vi "GV_YscaleDeletePoint.vi"(7 "Move?":bool, 8 "error in (no error)":errorcluster, 9 "Pos":cluster{"x":i16, "y":i16}, 10 "Plot in":picture, 11 "Gviewer in":refnum<class "Gviewer.lvclass">) -> (0 "error out":errorcluster, 2 "Plot out":picture, 3 "Gviewer out":refnum<class "Gviewer.lvclass">)   [LabVIEW 2020, in "Sgraph_lib_V1.lvlib" / "Gviewer.lvclass"]
doc: "Andre Koelewijn,11 aug 2021\n\nFocus Y-scale if selected"
uses:
  Gviewer.lvclass
  <vilib>/Utility/miscctls.llb/LVPoint32TypeDef.ctl
  Gviewer.lvclass/Gviewer.ctl
panel:
  in  "Coords":T1
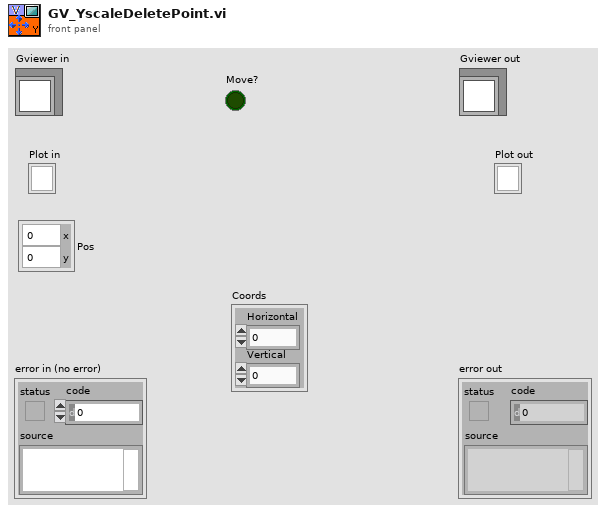
[diagram p1: front panel]
types:
  T1 = typedef "LVPoint32TypeDef.ctl" = cluster{"Horizontal":i32, "Vertical":i32}
  T2 = cluster{"left":i16, "top":i16, "right":i16, "bottom":i16}
  T3 = cluster{"Width":i16, "Style":enum32{"Solid", "Dash", "Dot", "DashDot", "DashDotDot"}}
  T4 = typedef "Sgraph_lib_V1.lvlib/Gviewer.lvclass/YgraphDef.ctl" = cluster{"Plot":i32, "X(%)":dbl}
  T5 = typedef "LVRectTypeDef.ctl" = cluster{"Left":i16, "Top":i16, "Right":i16, "Bottom":i16}
  T6 = cluster{"data":dbl[], "max":dbl[], "min":dbl[], "Status":u32[]}[]
  T7 = typedef "Sgraph_lib_V1.lvlib/Gviewer.lvclass/Typedef_SelProperties.ctl" = cluster{"Color":u32, "LineType":T8, "max":dbl, "min":dbl}
  T8 = typedef "Sgraph_lib_V1.lvlib/Gviewer.lvclass/Typedef_LineType.ctl" = enum16{"num_bare", "num_MinMax_Area", "num_MinMax_Lines", "num_MinMax_Forfor", "num_Max_Area", "num_Max_Line", "num_Max_Forfor", "num_Min_Area", "num_Min_Line", "num_Min_Fosfor", "Boolean_Line_01", "Boolean_Area_01", "Boolean_Fosfor_01", "Boolean_Line_TF", "Boolean_Area_TF", "Boolean_Fosfor_TF", "Boolean_OnOff_Line", "Boolean_OnOff_Area", "Boolean_OnOff_Fosfor", "Boolean_spare", "StringEvent_Line", "StringEvent_TimeLine"}
  T9 = cluster{"data":dbl[], "max":dbl[], "min":dbl[], "Status":u32[]}
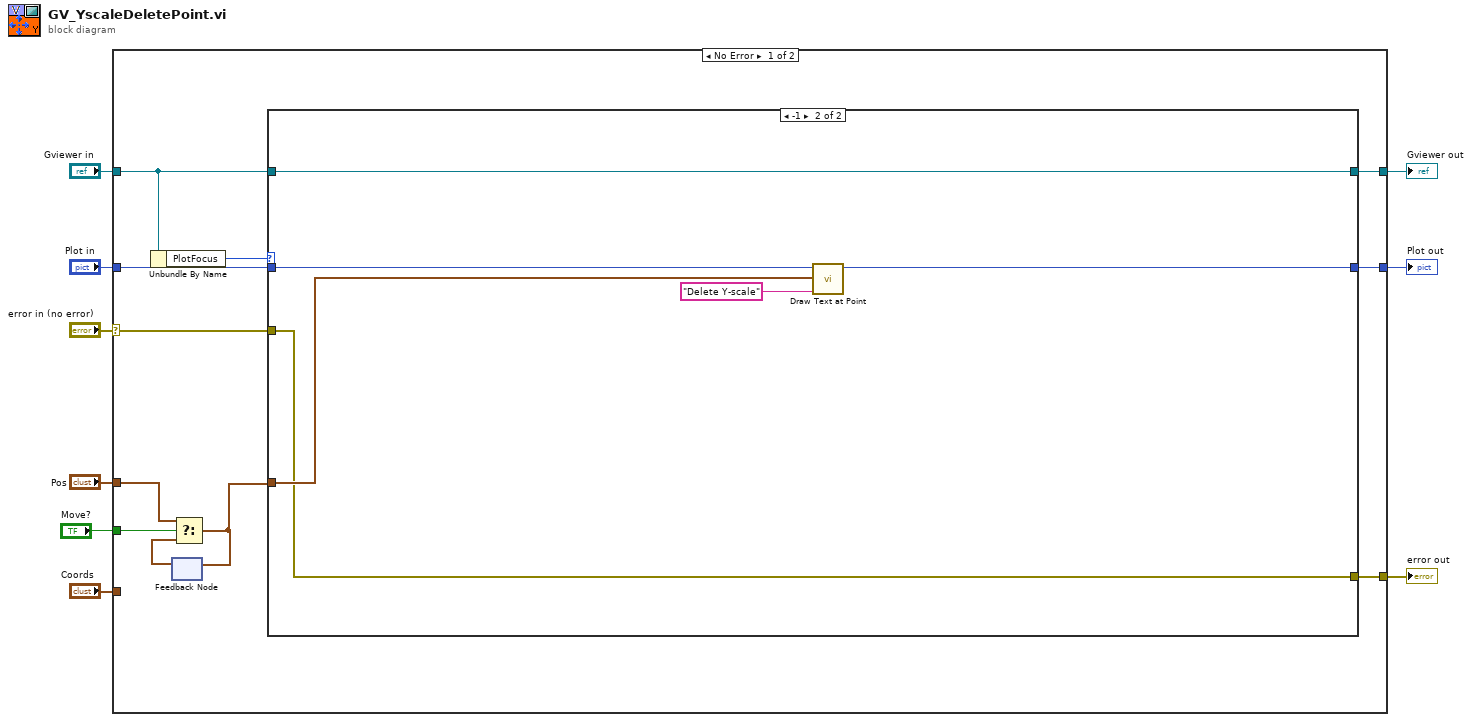
[diagram p0: block diagram]
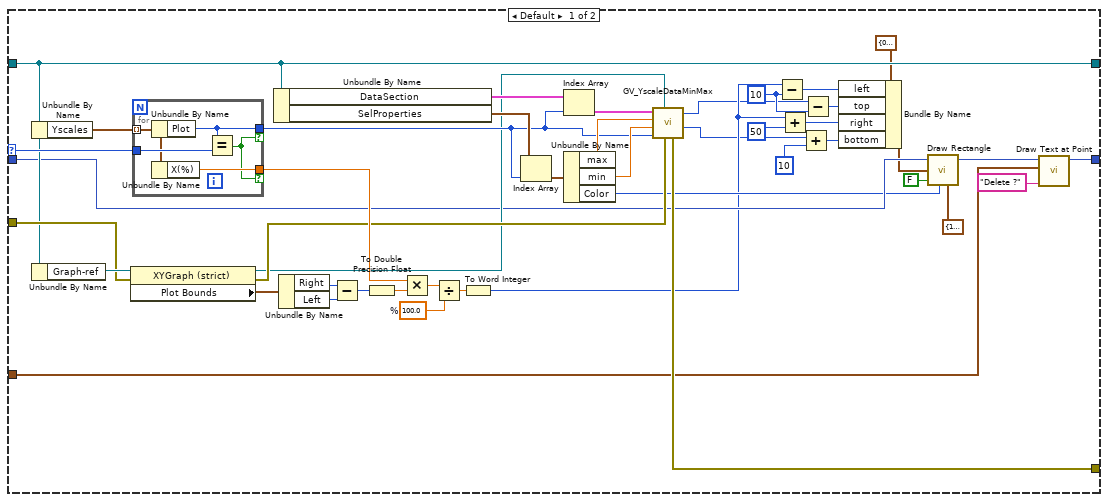
[diagram p2: hidden frame]
diagram:
  n1 = case shown="No Error" "error in (no error)" {
    selector: "error in (no error)" -> [w18 w77]
    tunnel: [w15 w77] -> w8
    tunnel: [w17 w76] -> w6
    tunnel: "Gviewer in" -> [w19 w76]
    tunnel: "Coords" -> [_ _]
    tunnel: [w16 _] -> w4
    tunnel: "Pos" -> [w10 _]
    tunnel: "Plot in" -> [w14 _]
    tunnel: "Move?" -> [w13 _]
    frame No Error {
      n2 = Unbundle By Name(w19) -> ("PlotFocus"=w20:i32)
      n3 = feedback #1() -> (w12:cluster{"x":i16, "y":i16})  [unwired: 1 in]
      n4 = Select(t=w10, s=w13, f=w12) -> (s? t:f=w11:cluster{"x":i16, "y":i16})
      n5 = feedback-in #1(w11) -> ()
      n6 = case shown="-1" w20 {
        selector: w20 -> [w63 _]
        tunnel: [w37 w75] -> w16
        tunnel: w11 -> [w36 w73]
        tunnel: [w43 w72] -> w15
        tunnel: w18 -> [w53 w72]
        tunnel: w19 -> [w50 w71]
        tunnel: [w50 w71] -> w17
        tunnel: w14 -> [w40 w70]
        frame Default {
          w27 = i16 10 ("y")
          w59 = 100.0  # %
          n7 = Unbundle By Name(w50) -> ("Yscales"=w64:T4[])
          n8 = Unbundle By Name(w50) -> ("Graph-ref"=w54:refnum<vi>)
          n9 = property class="XYGraph (strict)"(reference=w54, error in=w53) -> (reference out=w41:refnum<vi>, error out=w44:errorcluster, "Plot Bounds"=w52:T5)
          n10 = for {
            tunnel: w64 -> [w67] mode=indexing
            tunnel: [w68] -> w42 if=w65
            tunnel: w63 -> [w69]
            tunnel: [w66] -> w56 if=w65
            n11 = Unbundle By Name(w67) -> ("Plot"=w68:i32)
            n12 = Unbundle By Name(w67) -> ("X(%)"=w66:dbl)
            n13 = Equal?(x=w68, y=w69) -> (x = y?=w65:bool)
          }
          n14 = Unbundle By Name(w50) -> ("DataSection"=w48:T6, "SelProperties"=w49:T7[])
          n15 = Unbundle By Name(w52) -> ("Right"=w62:i16, "Left"=w61:i16)
          n16 = Subtract(x=w62, y=w61) -> (x-y=w55:i16)
          n17 = To Double Precision Float(number=w55) -> (double precision float=w57:dbl)
          n18 = Multiply(x=w56, y=w57) -> (x*y=w60:dbl)
          n19 = Divide(x=w60, y=w59) -> (x/y=w58:dbl)
          n20 = To Word Integer(number=w58) -> (16bit integer=w29:i16)
          n21 = Index Array(array=w49, index=w42) -> (element=w51:T7)
          n22 = Index Array(array=w48, index=w42) -> (element=w47:T9)
          n23 = Unbundle By Name(w51) -> ("max"=w46:dbl, "min"=w45:dbl, "Color"=w35:u32)
          n24 = call "GV_YscaleDataMinMax.vi"("error in (no error)"=w44, "Graph-ref"=w41, "Plot"=w42, "Scale-min"=w45, "Scale-max"=w46, "PAQ-data"=w47) -> ("Coord-min"=w21:i32, "Coord-max"=w22:i32, "error out"=w43:errorcluster)  [unwired: 1 in, 2 out]
          n25 = Subtract(x=w29, y=w27) -> (x-y=w30:i16)
          n26 = Add(x=w29, y=i16 50) -> (x+y=w25:i16)
          n27 = Add(x=w21, y=i16 10) -> (x+y=w23:i32)
          n28 = Subtract(x=w22, y=w27) -> (x-y=w26:i32)
          n29 = Bundle By Name(cluster=T2 {"left"=0, "top"=0, "right"=0, "bottom"=0} ("rect"), "left"=w30, "top"=w26, "right"=w25, "bottom"=w23) -> (w32:T2)
          n30 = call <vilib>:"Draw Rectangle.vi"("picture"=w40, "rect"=w32, "fill?(F)"=FALSE, "color(black)"=w35, "pen"=T3 {"Width"=1, "Style"=enum."Dot"}) -> ("new picture"=w38:picture)  [unwired: 4 in]
          n31 = call <vilib>:"Draw Text at Point.vi"("text"="Delete ?", "origin"=w36, "picture"=w38) -> ("new picture"=w37:picture)  [unwired: 7 in, 1 out]
        }
        frame -1 {
          n32 = call <vilib>:"Draw Text at Point.vi"("text"="Delete Y-scale", "origin"=w73, "picture"=w70) -> ("new picture"=w75:picture)  [unwired: 7 in, 1 out]
        }
      }
    }
    frame Error {
    }
  }
  "error out" <- w8
  "Gviewer out" <- w6
  "Plot out" <- w4
